vi "LampControl.vi"(8 "error in (no error)":errorcluster caption="错误输入（无错误）", 10 "ÈýÉ«Ÿô î‘B":T1, 11 "DevControl 输入":refnum<class "DevControl.lvclass"> caption="DNL_LabVIEW Object in") -> (0 "error out":errorcluster caption="错误输出", 3 "DevControl 输出":refnum<class "DevControl.lvclass"> caption="DNL_LabVIEW Object out")   [LabVIEW 2012, in "DevControl.lvclass"]
uses:
  DevControl.lvclass
  SupportVi/LampState.ctl
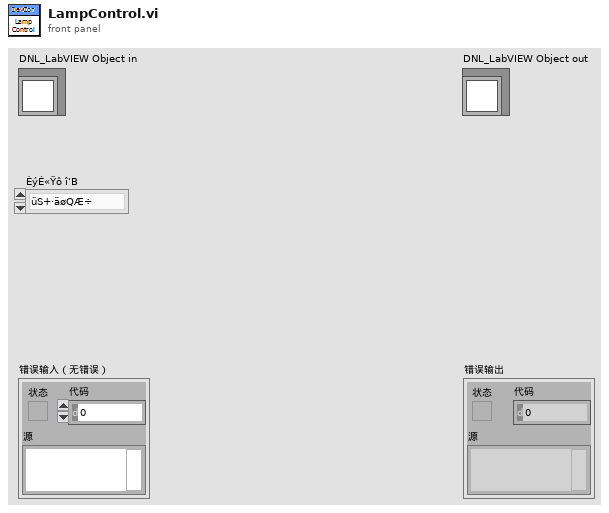
[diagram p1: front panel]
types:
  T1 = typedef "DevControl.lvclass/LampState.ctl" = enum16{"üS+·äøQÆ÷", "¼t+·äøQÆ÷", "·äøQÆ÷", "È«œç", "全亮", "üS", "¾G", "¼t"}
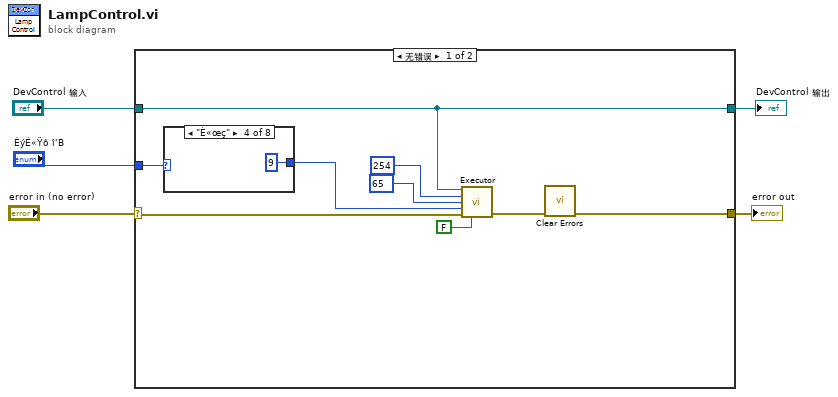
[diagram p0: block diagram]
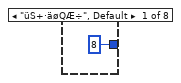
[diagram p2: hidden frame]
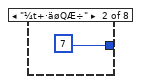
[diagram p3: hidden frame]
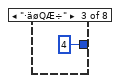
[diagram p4: hidden frame]
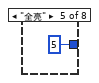
[diagram p5: hidden frame]
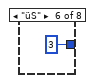
[diagram p6: hidden frame]
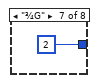
[diagram p7: hidden frame]
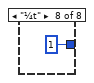
[diagram p8: hidden frame]
diagram:
  n1 = case shown="无错误" "error in (no error)" {
    selector: "error in (no error)" -> [w14 w24]
    tunnel: [w6 w24] -> w4
    tunnel: [w13 w23] -> w2
    tunnel: "DevControl 输入" -> [w13 w23]
    tunnel: "ÈýÉ«Ÿô î‘B" -> [w10 _]
    frame No Error {
      n2 = case shown="\"È«œç\"" w10 {
        tunnel: [u8 8 u8 7 u8 4 u8 9 u8 5 u8 3 u8 2 u8 1] -> w9
        frame "üS+·äøQÆ÷", Default {
        }
        frame "¼t+·äøQÆ÷" {
        }
        frame "·äøQÆ÷" {
        }
        frame "È«œç" {
        }
        frame "全亮" {
        }
        frame "üS" {
        }
        frame "¾G" {
        }
        frame "¼t" {
        }
      }
      n3 = call-dynamic "Executor.vi"("DevControl 输入"=w13, "Addr"=u8 254, "DevCmd"=u8 65, "Data"=w9, "error in (no error)"=w14, "ChkDat?"=FALSE) -> ("error out"=w7:errorcluster)  [unwired: 7 in, 2 out]
      n4 = call <vilib>:"Clear Errors.vi"("error in (no error)"=w7) -> ("error out"=w6:errorcluster)  [unwired: 6 in]
    }
    frame Error {
    }
  }
  "error out" <- w4
  "DevControl 输出" <- w2
